vi "FPGA fast output.vi"(6 "underflow warning level":u32, 7 "flush queue?":bool, 8 "fast queue idle in":bool, 10 "9269 Output Enabled":bool, 11 "fast output in":T1) -> (0 "fast queue idle out":bool, 2 "underflow warning":bool, 3 "fast output out":T1)   [LabVIEW 2018]
uses:
  <vilib>/rvi/Emulation/niFpgaGetClockAttributes.vi
  <vilib>/rvi/Emulation/niFpgaSctlEmulationGetInTimedLoop.vi
  <vilib>/rvi/Emulation/niFpgaEmulationReportErrorSimple.vi
  <vilib>/rvi/interface/RandomDataEmulation/niFpgaRandomDataHandleErrors.vi
  <vilib>/rvi/DataTransferAndStorage/Container/Common/niFpgaContainerExecOnDevCompGetState.vi
  <vilib>/rvi/Emulation/niFpgaEmulationIsFPGAContextNoSignature.vi
  <vilib>/rvi/errors/niFpgaSetErrorForExecOnDevCompSimple.vi
  <vilib>/rvi/eio/common/nirviEmuReportErrorAndStop.vi
  <vilib>/rvi/DataTransferAndStorage/Container/Common/niFpgaContainerGetUniqueNameForEmu.vi
  <vilib>/rvi/FIFO/Fifo_Resource/nirvififoEmulationSetSize.vi
  <vilib>/rvi/FIFO/Fifo_Resource/nirviFifoEmulationQueueMgr.vi
  <instcachedir>/0/nirviFifoEmulationQueueMgr_E5CAEC123FF24DC58D834DCA3CDAA9B5.lvgen/nirviFifoEmulationQueueMgr_E5CAEC123FF24DC58D834DCA3CDAA9B5_001.vi
  <vilib>/rvi/FIFO/Fifo_Resource/nirvififoEmulationDetermineInputValidOut.vi
  <vilib>/rvi/FIFO/Fifo_Resource/nirvififoEmulationCreateLock.vi
  <vilib>/rvi/Emulation/niFpgaProcessEmulError.vi
  <vilib>/rvi/FIFO/Fifo_Resource/nirvififoEmulationObtainLock.vi
  <vilib>/rvi/FIFO/Fifo_Resource/nirvififoEmulationReleaseLock.vi
  <vilib>/rvi/occurrence/nirviWaitOnOccurrenceBase.vi
  <vilib>/rvi/errors/nirviReportUnexpectedCaseInternalError.vi
  <vilib>/rvi/errors/nirviReportUnexpectedCaseInternalError (U32).vi
  <vilib>/Utility/error.llb/Clear Errors.vi
  <vilib>/rvi/Emulation/niFpgaCriticalErrorInLSC.vi
  <vilib>/rvi/eio/common/nirviEmuTemplateMethod_errors.vi
  <vilib>/rvi/DataTransferAndStorage/Container/XNode/niFpgaContainer.xnode
  <vilib>/rvi/interface/RandomDataEmulation/nirviRandomDataFpgaReadWriteTemplate.vi
  <vilib>/rvi/FIFO/Fifo_Resource/niFpgaFifoEmulationRefIn.vi
  <vilib>/eio/EIONode/EIONode.xnode
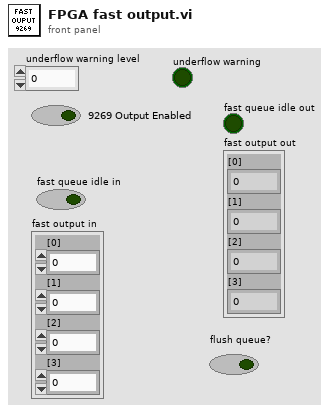
[diagram p1: front panel]
types:
  T1 = cluster{"[0]":fxp<+/-,20,5>, "[1]":fxp<+/-,20,5>, "[2]":fxp<+/-,20,5>, "[3]":fxp<+/-,20,5>}
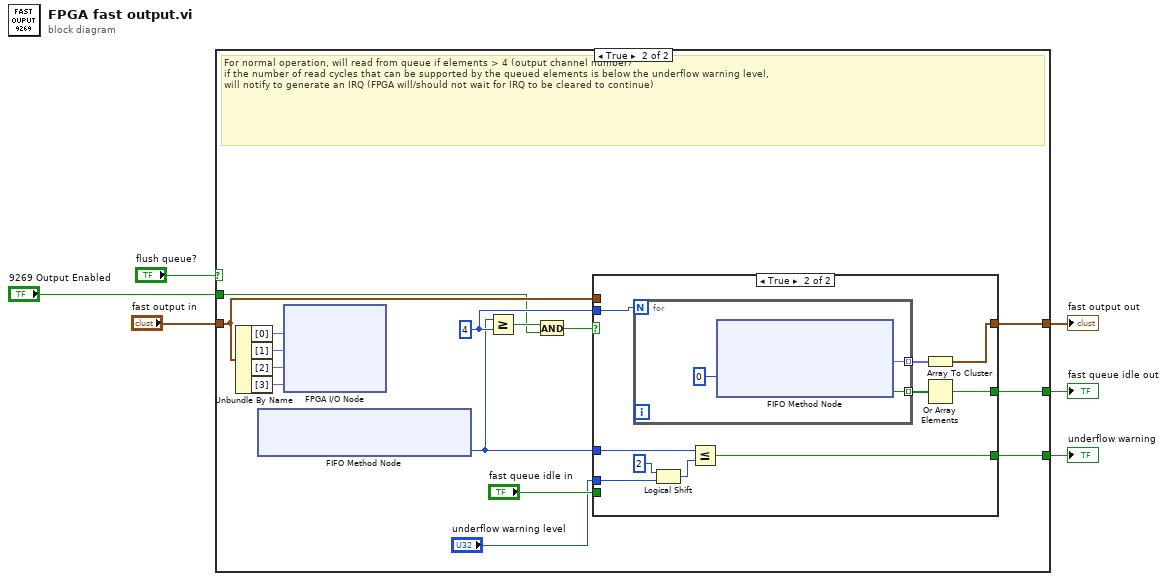
[diagram p0: block diagram]
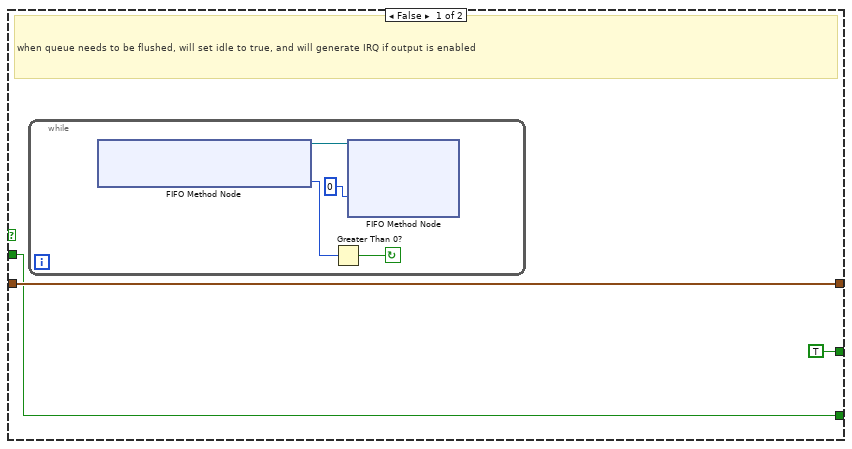
[diagram p2: hidden frame]
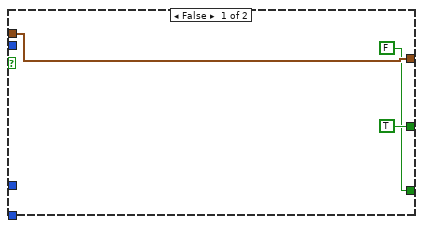
[diagram p3: hidden frame]
diagram:
  n1 = case shown="True" "flush queue?" {
    tunnel: [TRUE w28] -> w6
    tunnel: [w8 w27] -> w5
    tunnel: [w7 w16] -> w4
    tunnel: "fast output in" -> [w8 w15]
    tunnel: "9269 Output Enabled" -> [w7 w14]
    frame False {
      # "when queue needs to be flushed, will set idle to true, and will generate IRQ if output is enabled"
      n2 = while {
        stop <- w12 continue-if-true
        n3 = xnode ("FIFO Method Node")() -> ("Number of Elements to Read"=w13:u32, "FIFO Out"=w11:refnum<k21>)  [unwired: 1 in]
        n4 = Greater Than 0?(x=w13) -> (x > 0?=w12:bool)
        n5 = xnode ("FIFO Method Node")("Timeout"=0, "FIFO In"=w11) -> ()  [unwired: 3 out]
      }
    }
    frame True {
      w24 = u32 4 ("y")
      # "For normal operation, will read from queue if elements > 4 (output channel number)\nif the number of read cycles that can be supported by the queued elements is below the underflow warning level, \nwill notify to generate an IRQ (FPGA will/should not wait for IRQ to be cleared to continue)"
      n6 = Unbundle By Name(w15) -> ("[0]"=w22:fxp<+/-,20,5>, "[1]"=w21:fxp<+/-,20,5>, "[2]"=w20:fxp<+/-,20,5>, "[3]"=w19:fxp<+/-,20,5>)
      n7 = xnode ("FIFO Method Node")() -> ("Number of Elements to Read"=w18:u32)  [unwired: 1 in, 1 out]
      n8 = xnode "FPGA I/O Node"("Mod1/AO0"=w22, "Mod1/AO1"=w21, "Mod1/AO2"=w20, "Mod1/AO3"=w19) -> ()  [unwired: 4 in, 4 out]
      n9 = Greater Or Equal?(x=w18, y=w24) -> (x >= y?=w25:bool)
      n10 = And(x=w25, y=w14) -> (x .and. y?=w23:bool)
      n11 = case shown="True" w23 {
        tunnel: w24 -> [_ w37]
        tunnel: [TRUE w40] -> w28
        tunnel: [w31 w38] -> w27
        tunnel: w15 -> [w31 _]
        tunnel: "fast queue idle in" -> [_ _]
        tunnel: w18 -> [_ w36]
        tunnel: "underflow warning level" -> [_ w34]
        tunnel: [FALSE w35] -> w16
        frame False {
        }
        frame True {
          n12 = for {
            N: w37 -> [_]
            tunnel: [w43] -> w41 mode=indexing
            tunnel: [w42] -> w39 mode=indexing
            n13 = xnode ("FIFO Method Node")("Timeout"=0) -> ("Element"=w42:fxp<+/-,20,5>, "Timed Out?"=w43:bool)  [unwired: 1 in, 1 out]
          }
          n14 = Logical Shift(y=i16 2, x=w34) -> (x << y=w32:u32)
          n15 = Less Or Equal?(x=w36, y=w32) -> (x <= y?=w35:bool)
          n16 = Array To Cluster(array=w39) -> (cluster=w38:T1)
          n17 = Or Array Elements(Boolean array=w41) -> (logical OR=w40:bool)
        }
      }
    }
  }
  "fast queue idle out" <- w6
  "fast output out" <- w5
  "underflow warning" <- w4
